vi "logPacket.vi"(0 "file path (dialog if empty)":path, 5 "altitude":i32, 7 "internal temp":i32, 9 "external temp":i32, 11 "humidity":i32) -> ()   [LabVIEW 2012]
uses:
  <vilib>/Utility/file.llb/Write To Spreadsheet File (string).vi
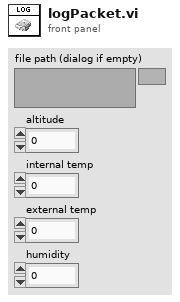
[diagram p1: front panel]
types:
  T1 = enum16{"open", "replace", "create", "open or create", "replace or create", "replace or create with confirmation"}
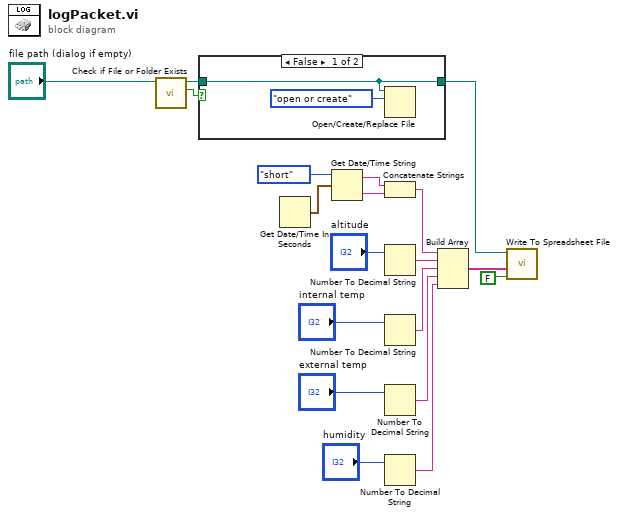
[diagram p0: block diagram]
diagram:
  n1 = call <vilib>:"Check if File or Folder Exists.vi"("path"="file path (dialog if empty)") -> ("file or folder exists?"=w3:bool, "dup path"=w4:path)  [unwired: 8 in, 1 out]
  n2 = case shown="False" w3 {
    tunnel: w4 -> [w20 w22]
    tunnel: [w20 w22] -> w1
    frame False {
      n3 = Open/Create/Replace File(file path (use dialog)=w20, operation (0:open)=T1."open or create") -> ()  [unwired: 4 in, 3 out]
    }
    frame True {
    }
  }
  n4 = Get Date/Time In Seconds() -> (seconds since 1Jan1904=w16:timestamp)
  n5 = Get Date/Time String(date format (0)=enum16{"short", "long", "abbreviated"}."short", seconds (now)=w16) -> (date string=w18:string, time string=w19:string)  [unwired: 1 in]
  n6 = Concatenate Strings(w18, w19) -> (w15:string)
  n7 = Number To Decimal String(number="altitude") -> (decimal integer string=w13:string)  [unwired: 1 in]
  n8 = Number To Decimal String(number="internal temp") -> (decimal integer string=w12:string)  [unwired: 1 in]
  n9 = Number To Decimal String(number="external temp") -> (decimal integer string=w11:string)  [unwired: 1 in]
  n10 = Number To Decimal String(number="humidity") -> (decimal integer string=w10:string)  [unwired: 1 in]
  n11 = Build Array(w15, w13, w12, w11, w10) -> (w2:string[])
  n12 = call-poly <vilib>:"Write To Spreadsheet File.vi"("append to file? (new file:F)"=FALSE, "1D data"=w2, "file path (dialog if empty)"=w1) -> ()  [unwired: 5 in, 1 out]
